vi "Check Next Trigger State (hybrid).vi"(8 "error in (no error)":errorcluster, 9 "Array of States LUT":variant[](array[variant]), 10 "States LUT (name -> boolean state)":variant, 11 "TriggerAction in":refnum<class "TriggerAction Q.lvclass">) -> (0 "error out":errorcluster, 2 "Trigger State":bool, 3 "TriggerAction out":refnum<class "TriggerAction Q.lvclass">)   [LabVIEW 2016, in "TriggerAction Q.lvclass"]
uses:
  <userlib>/Common Components/TriggerAction Q/TriggerAction Q/TriggerAction Q.lvclass
  <userlib>/Common Components/TriggerAction Q/TriggerAction Q/TriggerAction Q.lvclass/TriggerAction Q.ctl
  <userlib>/Common Components/TriggerAction Q/TriggerAction Q/Trigger Cluster.ctl
  <vilib>/Utility/error.llb/Error Cluster From Error Code.vi
  <vilib>/ErrorRing/Error Ring.xnode
  <vilib>/addons/_JKI.lib/Serialization/JSON/JKI JSON Serialization.lvlib
panel:
  # "System level states"
  # "States of each motion"
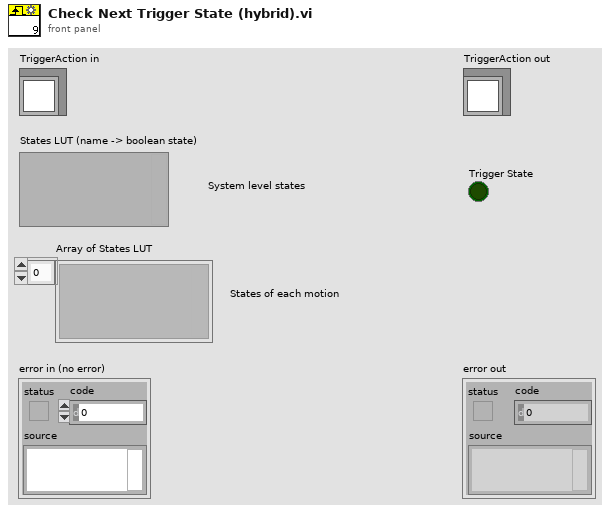
[diagram p1: front panel]
types:
  T1 = typedef "TriggerAction.lvclass/Element Data.ctl" = cluster{"Triggers":cluster{"Triggers for Array AND":string[]}[], "Actions":cluster{"Action Name":string, "Action Data":string}[]}
  T2 = typedef "TriggerAction Q.lvclass/Trigger Cluster.ctl" = cluster{"Index":u8, "State Name":string}
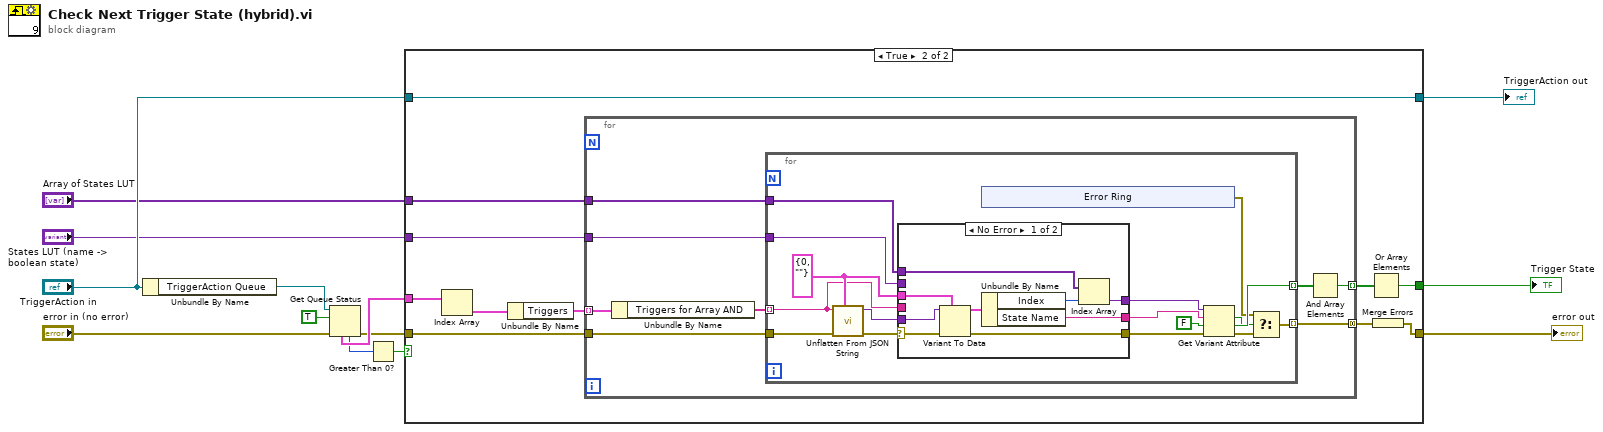
[diagram p0: block diagram]
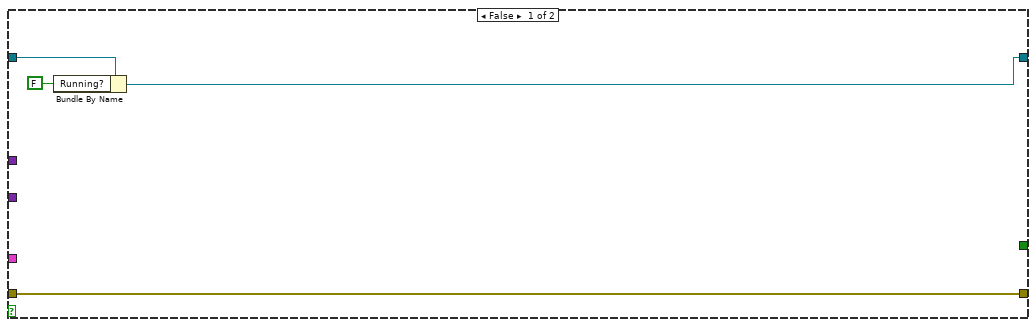
[diagram p2: hidden frame]
diagram:
  n1 = Unbundle By Name("TriggerAction in") -> ("TriggerAction Queue"=w13:refnum<queue>)
  n2 = Get Queue Status(queue=w13, return elements? (F)=TRUE, error in (no error)="error in (no error)") -> (error out=w4:errorcluster, # elements in queue=w9:i32, elements=w11:T1[])  [unwired: 5 out]
  n3 = Greater Than 0?(x=w9) -> (x > 0?=w8:bool)
  n4 = case shown="True" w8 {
    tunnel: w11 -> [_ w28]
    tunnel: "Array of States LUT" -> [_ w25]
    tunnel: [_ w23] -> w10
    tunnel: "TriggerAction in" -> [w17 w22]
    tunnel: [w15 w22] -> w6
    tunnel: w4 -> [w14 w21]
    tunnel: [w14 w19] -> w3
    tunnel: "States LUT (name -> boolean state)" -> [_ w18]
    frame False {
      n5 = Bundle By Name(cluster=w17, "Running?"=FALSE) -> (w15:refnum<class "TriggerAction Q.lvclass">)
    }
    frame True {
      n6 = Index Array(array=w28) -> (element=w27:T1)  [unwired: 1 in]
      n7 = Unbundle By Name(w27) -> ("Triggers"=w26:cluster{"Triggers for Array AND":string[]}[])
      n8 = for {
        tunnel: w26 -> [w35] mode=indexing
        tunnel: w25 -> [w36]
        tunnel: [w32] -> w24 mode=indexing
        tunnel: w21 -> [w31]
        tunnel: [w30] -> w20 mode=concatenating
        tunnel: w18 -> [w29]
        n9 = Unbundle By Name(w35) -> ("Triggers for Array AND"=w33:string[])
        n10 = for {
          tunnel: w36 -> [w52]
          tunnel: [w51] -> w34 mode=indexing
          tunnel: w33 -> [w37] mode=indexing
          tunnel: w31 -> [w47]
          tunnel: [w50] -> w30 mode=indexing
          tunnel: w29 -> [w38]
          w48 = T2 {"Index"=0, "State Name"=""} ("Cluster")
          n11 = call <vilib>:"Unflatten From JSON String.vi"("Type and Defaults"=w48, "error in (no error)"=w47, "JSON String"=w37) -> ("error out"=w39:errorcluster, "Variant"=w49:variant)  [unwired: 7 in]
          n12 = case shown="No Error" w39 {
            selector: w39 -> [w53 _]
            tunnel: w52 -> [w61 _]
            tunnel: w49 -> [w60 _]
            tunnel: w48 -> [w59 _]
            tunnel: [w57 w63] -> w42
            tunnel: [w55 w62] -> w41
            tunnel: [w54 _] -> w40
            tunnel: w38 -> [_ w63]
            tunnel: w37 -> [_ w62]
            frame No Error {
              n13 = Variant To Data(error in=w53, type=w59, Variant=w60) -> (data=w58:T2, error out=w54:errorcluster)
              n14 = Unbundle By Name(w58) -> ("Index"=w56:u8, "State Name"=w55:string)
              n15 = Index Array(array=w61, index=w56) -> (element=w57:variant)
            }
            frame Error {
            }
          }
          n16 = xnode "Error Ring"() -> ("error out"=w44:errorcluster)
          n17 = Get Variant Attribute(Variant=w42, name=w41, default value (empty Variant)=FALSE, error in=w40) -> (found=w45:bool, value=w51:bool, error out=w43:errorcluster)  [unwired: 1 out]
          n18 = Select(t=w44, s=w45, f=w43) -> (s? t:f=w50:errorcluster)
        }
        n19 = And Array Elements(Boolean array=w34) -> (logical AND=w32:bool)
      }
      n20 = Or Array Elements(Boolean array=w24) -> (logical OR=w23:bool)
      n21 = Merge Errors(w20) -> (w19:errorcluster)
    }
  }
  "error out" <- w3
  "TriggerAction out" <- w6
  "Trigger State" <- w10
